vi "Reset Range Limits.vi"(8 "error in (no error)":errorcluster, 11 "Numeric Data Type in":refnum<class "Numeric Data Type.lvclass">) -> (0 "error out":errorcluster, 3 "Numeric Data Type out":refnum<class "Numeric Data Type.lvclass">)   [LabVIEW 2018, in "Numeric Data Type.lvclass"]
uses:
  Numeric Data Type.lvclass
  Numeric Data Type.lvclass/Numeric Data Type.ctl
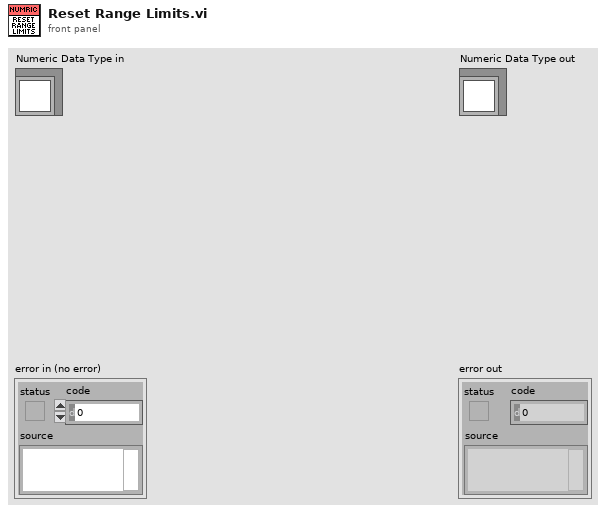
[diagram p1: front panel]
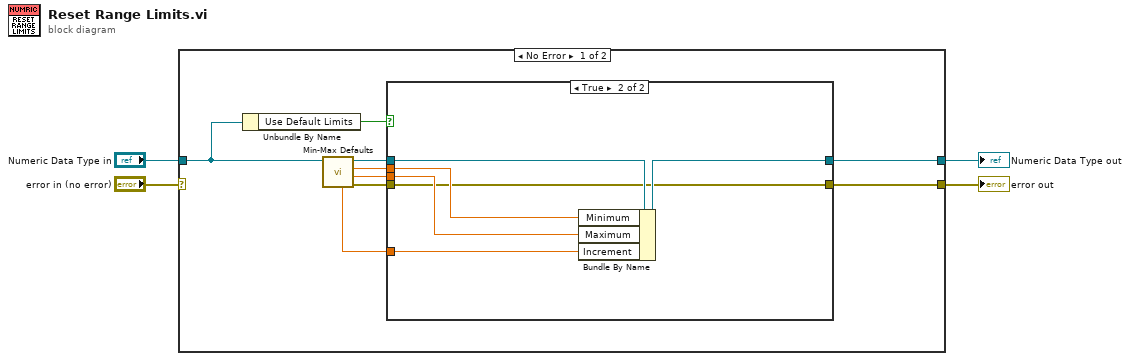
[diagram p0: block diagram]
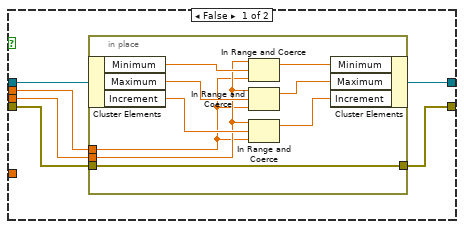
[diagram p2: hidden frame]
diagram:
  n1 = case shown="No Error" "error in (no error)" {
    selector: "error in (no error)" -> [_ w36]
    tunnel: [w13 w36] -> w3
    tunnel: [w12 w35] -> w1
    tunnel: "Numeric Data Type in" -> [w10 w35]
    frame No Error {
      n2 = Unbundle By Name(w10) -> ("Use Default Limits"=w11:bool)
      n3 = call "Min-Max Defaults.vi"("Numeric Data Type in"=w10) -> ("error out"=w5:errorcluster, "Maximum"=w7:dbl, "Minimum"=w8:dbl, "Numeric Data Type (dup)"=w9:refnum<class "Numeric Data Type.lvclass">, "Increment"=w6:dbl)  [unwired: 6 in]
      n4 = case shown="True" w11 {
        tunnel: [w14 w29] -> w13
        tunnel: [w18 w34] -> w12
        tunnel: w9 -> [w19 w33]
        tunnel: w8 -> [w17 w31]
        tunnel: w7 -> [w16 w30]
        tunnel: w6 -> [_ w32]
        tunnel: w5 -> [w15 w29]
        frame False {
          n5 = in-place {
            in-place-border: w16 -> [w25]
            in-place-border: w17 -> [w24]
            in-place-border: w15 -> [w20]
            in-place-border: [w20] -> w14
            n6 = in-place-cluster #1(w19) -> ("Minimum"=w28:dbl, "Maximum"=w27:dbl, "Increment"=w26:dbl)
            n7 = In Range and Coerce(upper limit=w25, x=w28, lower limit=w24) -> (coerced(x)=w23:dbl)  [unwired: 1 out]
            n8 = In Range and Coerce(upper limit=w25, x=w27, lower limit=w24) -> (coerced(x)=w22:dbl)  [unwired: 1 out]
            n9 = In Range and Coerce(upper limit=w25, x=w26, lower limit=w24) -> (coerced(x)=w21:dbl)  [unwired: 1 out]
            n10 = in-place-cluster #1("Minimum"=w23, "Maximum"=w22, "Increment"=w21) -> (w18:refnum<class "Numeric Data Type.lvclass">)
          }
        }
        frame True {
          n11 = Bundle By Name(cluster=w33, "Minimum"=w31, "Maximum"=w30, "Increment"=w32) -> (w34:refnum<class "Numeric Data Type.lvclass">)
        }
      }
    }
    frame Error {
    }
  }
  "error out" <- w3
  "Numeric Data Type out" <- w1
